vi "Search for Existing Error Code.vi"() -> ()   [LabVIEW 2015]
panel:
  out "Containing File":string
  out "Code Exists?":bool
  in  "Code Name":string
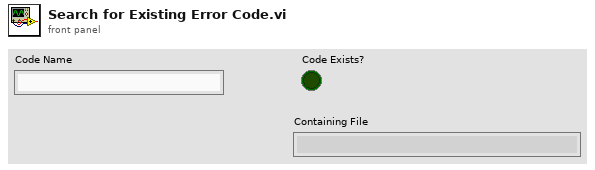
[diagram p1: front panel]
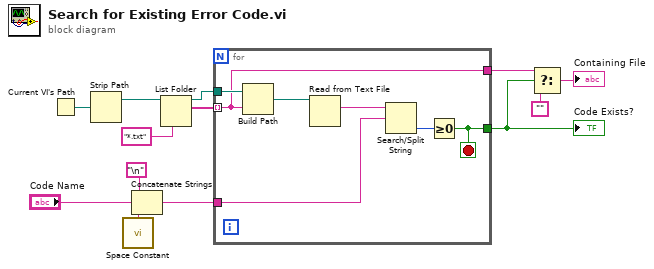
[diagram p0: block diagram]
diagram:
  n1 = Current VI's Path() -> (path=w13:path)
  n2 = Strip Path(path=w13) -> (stripped path=w12:path)  [unwired: 1 out]
  n3 = call <vilib>:"Space Constant.vi"() -> ("String"=w2:string)
  n4 = Concatenate Strings("\n", "Code Name", w2) -> (w3:string)
  n5 = List Folder(path=w12, pattern="*.txt") -> (path out=w9:path, filenames=w10:string[])  [unwired: 2 in, 2 out]
  n6 = for {
    tunnel: w10 -> [w14] mode=indexing
    tunnel: w9 -> [w20]
    tunnel: w3 -> [w17]
    tunnel: [w15] -> w7
    tunnel: [w14] -> w6
    stop <- w15 stop-if-true
    n7 = Build Path(base path=w20, name or relative path=w14) -> (appended path=w19:path)
    n8 = Read from Text File(file (use dialog)=w19) -> (text=w18:string)  [unwired: 3 in, 3 out]
    n9 = Search/Split String(string=w18, search string/char (-)=w17) -> (offset of match=w16:i32)  [unwired: 1 in, 2 out]
    n10 = Greater Or Equal To 0?(x=w16) -> (x >= 0?=w15:bool)
  }
  "Code Exists?" <- w7
  n11 = Select(t=w6, s=w7, f="") -> (s? t:f=→"Containing File":string)
